vi "Load DAC Configuration.vi"(8 "error in":errorcluster, 10 "Config File refnum in":T1, 11 "DAC LN2 Temp in":refnum<class "DAC LN2 Temp.lvclass">) -> (0 "error out":errorcluster, 2 "Config File refnum out":T1, 3 "DAC LN2 Temp out":refnum<class "DAC LN2 Temp.lvclass">)   [LabVIEW 2019, in "DAC.lvlib" / "DAC LN2 Temp.lvclass"]
uses:
  DAC LN2 Temp.lvclass
  C:/Users/krio/Documents/LV_Projects/test-stand/App/DAC/DAC.lvclass
  <vilib>/Utility/config.llb/Config Data RefNum.ctl
  DAC.lvclass/DAC.ctl
  DAC LN2 Temp.lvclass/DAC LN2 Temp.ctl
  <vilib>/Utility/config.llb/Read Key (String).vi
  <vilib>/Utility/config.llb/Read Key (Double).vi
  DAC.lvclass
  <vilib>/Utility/config.llb/NI_LVConfig.lvlib
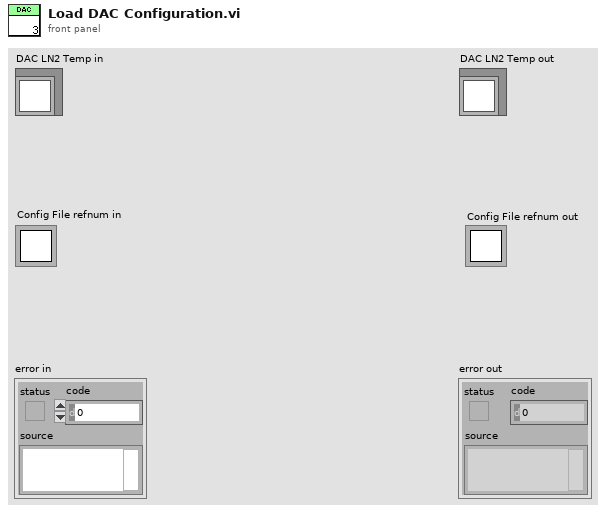
[diagram p1: front panel]
types:
  T1 = typedef "NI_LVConfig.lvlib/Config Data RefNum.ctl" = refnum<k1>
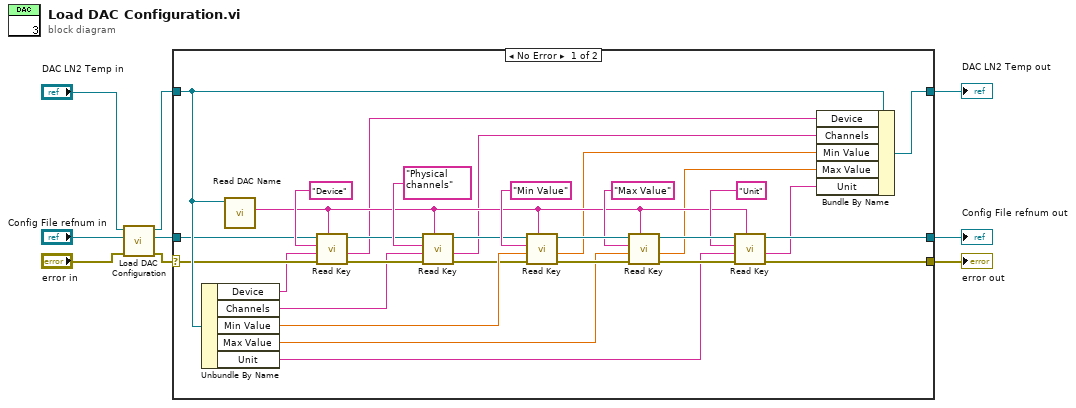
[diagram p0: block diagram]
diagram:
  n1 = call-parent "Load DAC Configuration.vi"("error in"="error in", "Config File refnum in"="Config File refnum in", "DAC in"="DAC LN2 Temp in") -> ("error out"=w4:errorcluster, "Config File refnum out"=w5:T1, "DAC out"=w6:refnum<class "DAC LN2 Temp.lvclass">)  [unwired: 6 in]
  n2 = case shown="No Error" w4 {
    selector: w4 -> [w21 w42]
    tunnel: [w32 w42] -> w1
    tunnel: [w30 w41] -> w3
    tunnel: w6 -> [w29 w41]
    tunnel: w5 -> [w22 w40]
    tunnel: [w31 w40] -> w2
    frame No Error {
      n3 = Unbundle By Name(w29) -> ("Device"=w17:string, "Channels"=w15:string, "Min Value"=w28:dbl, "Max Value"=w27:dbl, "Unit"=w26:string)
      n4 = call "Read DAC Name.vi"("DAC in"=w29) -> ("DAC Name"=w16:string)  [unwired: 8 in, 2 out]
      n5 = call-poly <vilib>:"Read Key.vi"("section"=w16, "error in (no error)"=w21, "default value"=w17, "key"="Device", "refnum"=w22) -> ("error out"=w20:errorcluster, "value"=w14:string, "refnum out"=w23:T1)  [unwired: 3 in, 1 out]
      n6 = call-poly <vilib>:"Read Key.vi"("section"=w16, "error in (no error)"=w20, "default value"=w15, "key"="Physical channels", "refnum"=w23) -> ("error out"=w18:errorcluster, "value"=w13:string, "refnum out"=w19:T1)  [unwired: 3 in, 1 out]
      n7 = call-poly <vilib>:"Read Key.vi"("section"=w16, "error in (no error)"=w18, "default value"=w28, "key"="Min Value", "refnum"=w19) -> ("error out"=w37:errorcluster, "value"=w12:dbl, "refnum out"=w39:T1)  [unwired: 3 in, 1 out]
      n8 = call-poly <vilib>:"Read Key.vi"("section"=w16, "error in (no error)"=w37, "default value"=w27, "key"="Max Value", "refnum"=w39) -> ("error out"=w36:errorcluster, "value"=w11:dbl, "refnum out"=w38:T1)  [unwired: 3 in, 1 out]
      n9 = call-poly <vilib>:"Read Key.vi"("section"=w16, "error in (no error)"=w36, "default value"=w26, "key"="Unit", "refnum"=w38) -> ("error out"=w32:errorcluster, "value"=w10:string, "refnum out"=w31:T1)  [unwired: 3 in, 1 out]
      n10 = Bundle By Name(cluster=w29, "Device"=w14, "Channels"=w13, "Min Value"=w12, "Max Value"=w11, "Unit"=w10) -> (w30:refnum<class "DAC LN2 Temp.lvclass">)
    }
    frame Error {
    }
  }
  "error out" <- w1
  "DAC LN2 Temp out" <- w3
  "Config File refnum out" <- w2
